vi "Launch_HMI.vi"(8 "error in (no error)":errorcluster caption="entrée d'erreur (pas d'erreur)", 11 "Class Popup (Default) en entrée":refnum<class "Popup Autotest (Default).lvclass">) -> (0 "error out":errorcluster caption="sortie d'erreur", 3 "Class Popup (Default) en sortie":refnum<class "Popup Autotest (Default).lvclass">)   [LabVIEW 2020, in "Library Instrument & Equipement.lvlib" / "Library Popup.lvlib" / "Popup Autotest (Default).lvclass"]
uses:
  Popup Autotest (Default).lvclass
  Class Popup (Main)/Class Popup (Main).lvclass
  Popup Autotest (Default).lvclass/Popup Autotest (Default).ctl
panel:
  in  "code":i32
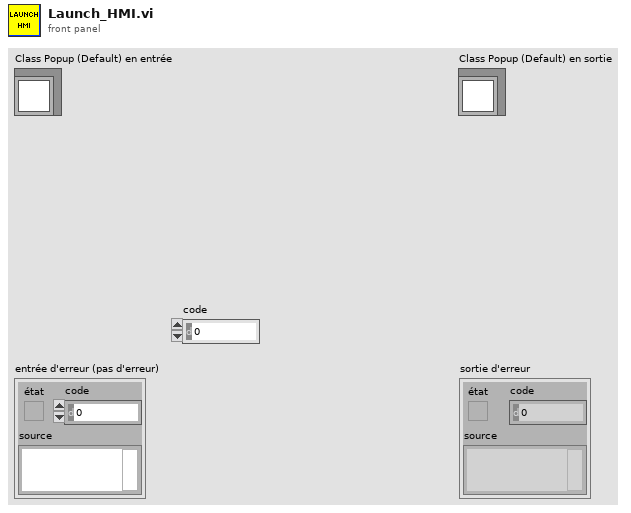
[diagram p1: front panel]
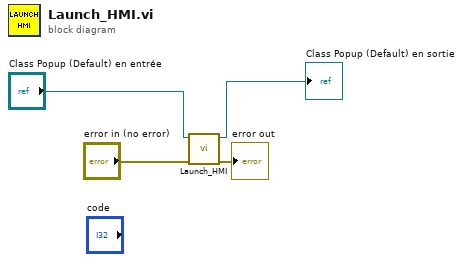
[diagram p0: block diagram]
diagram:
  n1 = call-parent "Launch_HMI.vi"("error in (no error)"="error in (no error)", "Class Popup (Default) en entrée"="Class Popup (Default) en entrée") -> ("error out"=→"error out":errorcluster, "Class Popup (Default) en sortie"=→"Class Popup (Default) en sortie":refnum<class "Popup Autotest (Default).lvclass">)  [unwired: 8 in]
